vi "Read Admin Enable.vi"(4 "Close 2":bool, 8 "error in (no error)":errorcluster, 11 "Masterv2 in":refnum<class "Masterv2.lvclass">) -> (0 "error out":errorcluster, 1 "Boolean":bool, 3 "Masterv2 out":refnum<class "Masterv2.lvclass">, 5 "Admin Enable":bool, 6 "User Enable":bool, 7 "Programmer Enable":bool)   [LabVIEW 2014, in "Main Libraryv2.lvlib" / "Masterv2.lvclass"]
uses:
  Master/Masterv2.lvclass
panel:
  in  "DEL 2":bool
  in  "1 2":bool
  in  "2 2":bool
  in  "3 2":bool
  in  "4 2":bool
  in  "5 2":bool
  in  "6 2":bool
  in  "7 2":bool
  in  "8 2":bool
  in  "9 2":bool
  in  "0 2":bool
  in  "Enter 2":bool
  out "Login PWD 2":string
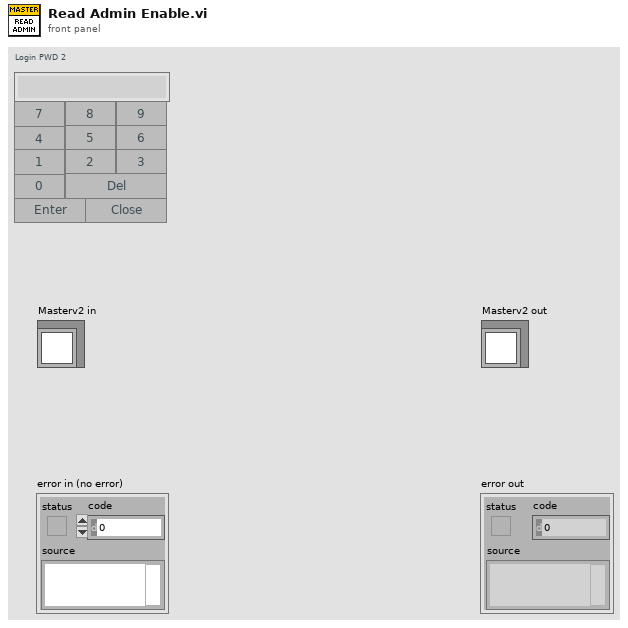
[diagram p1: front panel]
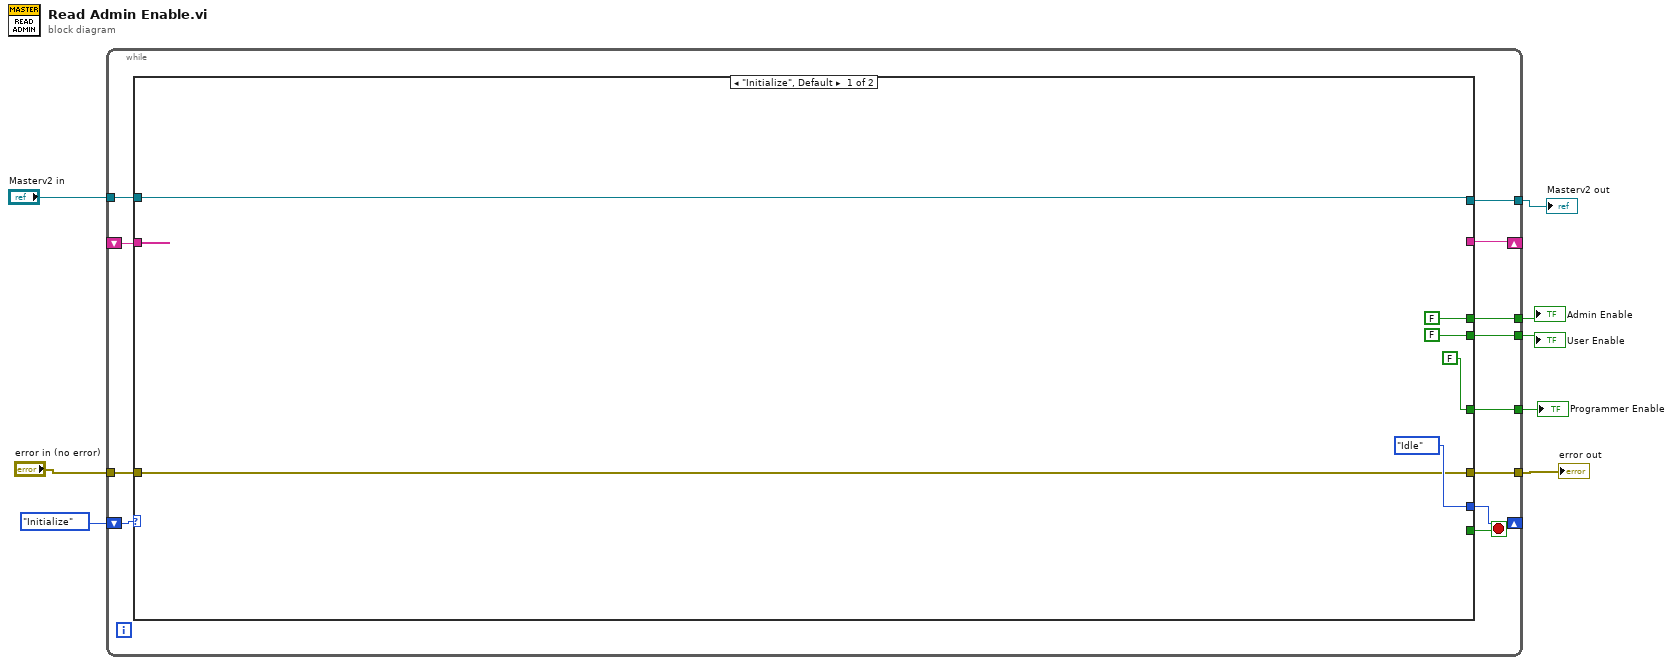
[diagram p0: block diagram]
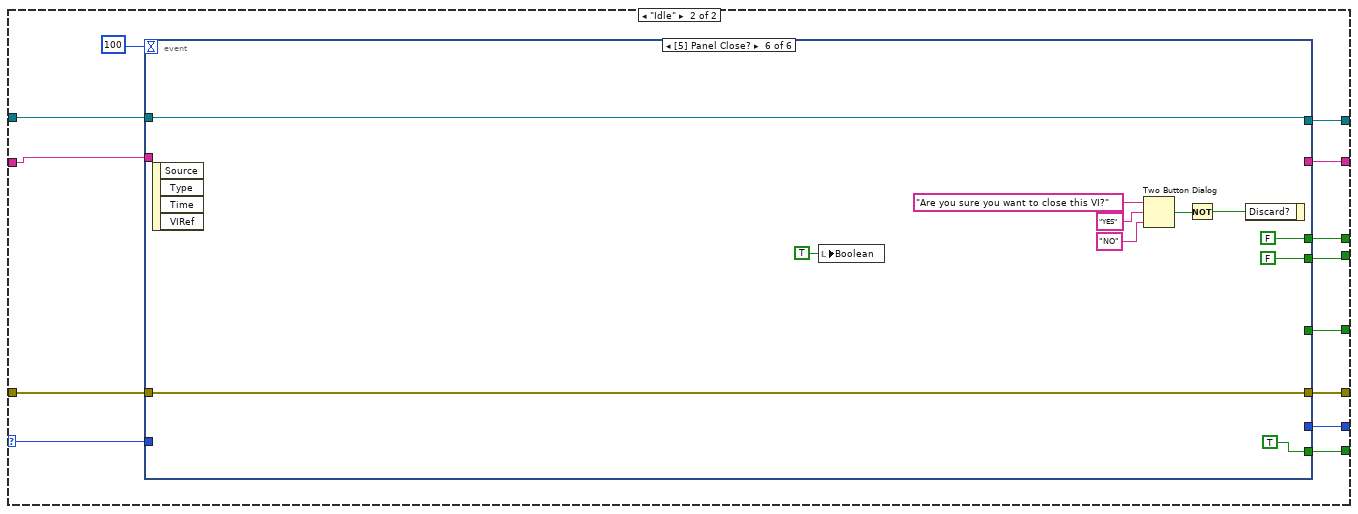
[diagram p2: hidden frame]
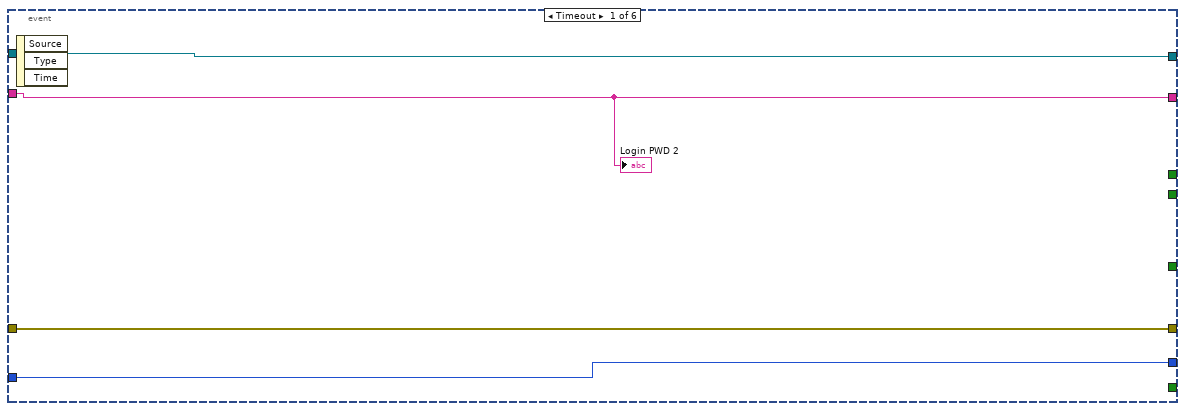
[diagram p3: hidden frame]
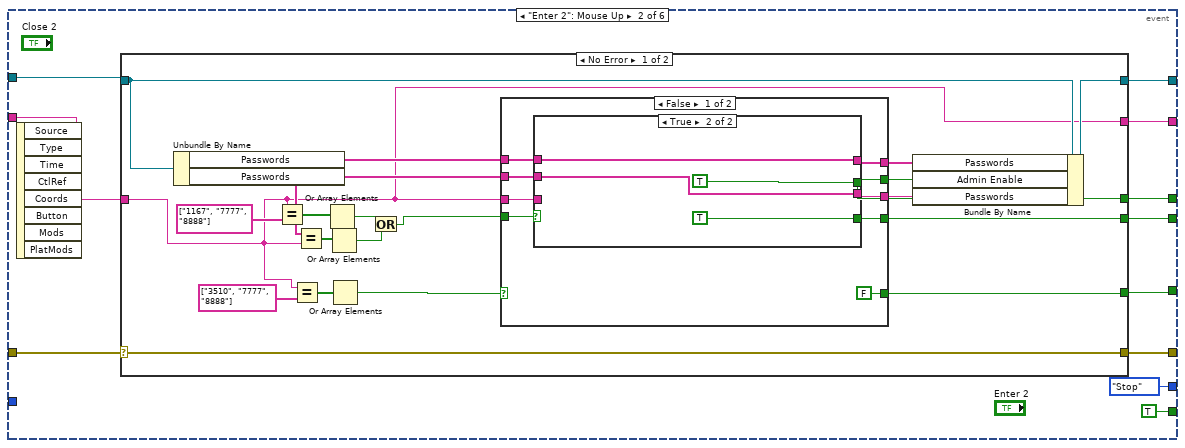
[diagram p4: hidden frame]
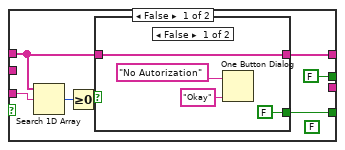
[diagram p5: hidden frame]
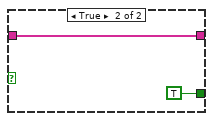
[diagram p6: hidden frame]
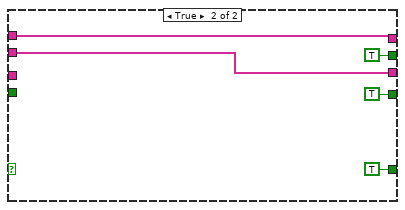
[diagram p7: hidden frame]
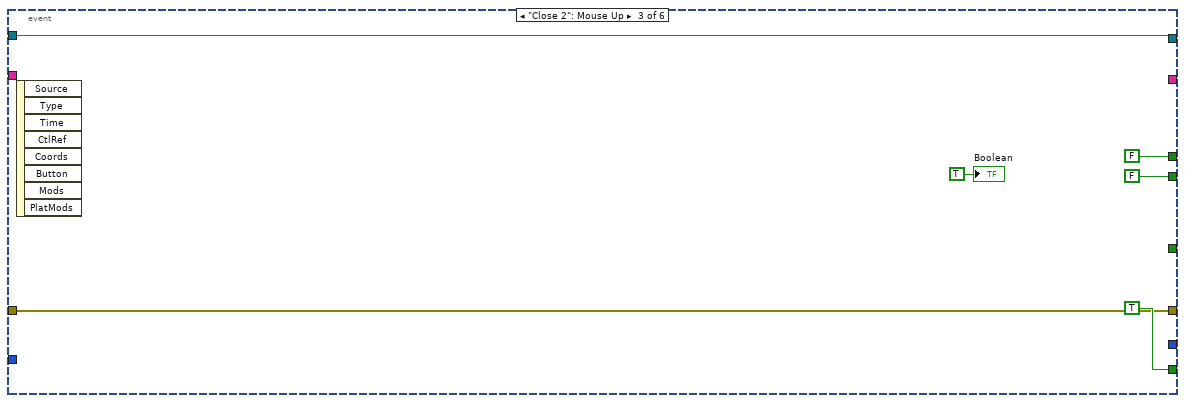
[diagram p9: hidden frame]
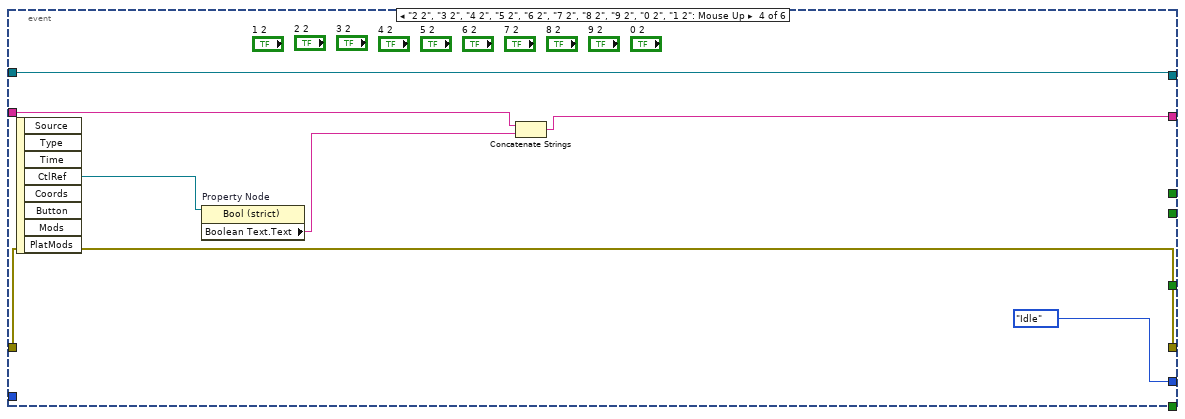
[diagram p10: hidden frame]
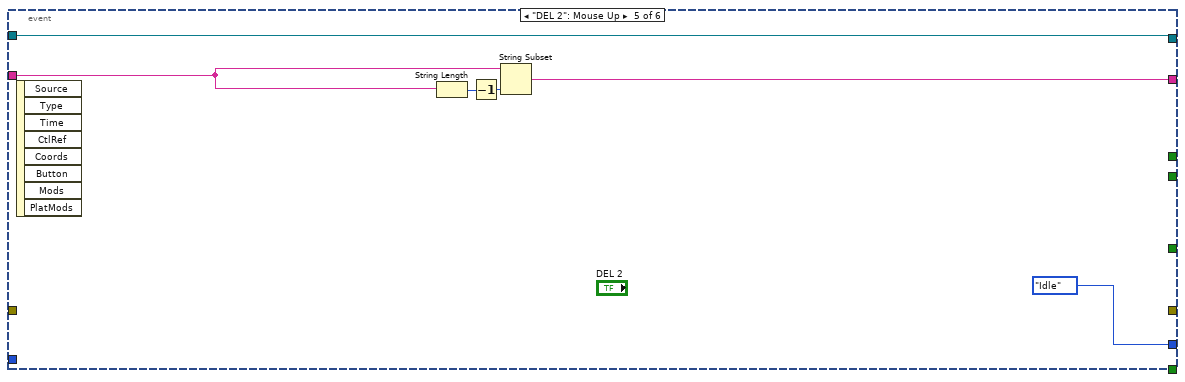
[diagram p11: hidden frame]
diagram:
  n1 = while {
    tunnel: "Masterv2 in" -> [w20]
    tunnel: "error in (no error)" -> [w19]
    tunnel: [w18] -> w2
    tunnel: [w17] -> w8
    tunnel: [w16] -> w7
    tunnel: [w15] -> w1
    shift-right: [w13] -> _
    shift-left: enum16{"Initialize", "Idle", "Stop"}."Initialize" -> [w14]
    shift-right: [w10] -> _
    shift-left: _ -> [w11]
    tunnel: [w9] -> w5
    stop <- w12 stop-if-true
    n2 = case shown="\"Initialize\", Default" w14 {
      selector: w14 -> [_ w32]
      tunnel: w20 -> [w24 w39]
      tunnel: w19 -> [w25 w38]
      tunnel: [w24 w37] -> w18
      tunnel: [FALSE ("Admin Enable") w36] -> w17
      tunnel: [FALSE ("User Enable") w35] -> w16
      tunnel: [w25 w34] -> w15
      tunnel: [enum16{"Initialize", "Idle", "Stop"}."Idle" w33] -> w13
      tunnel: [_ w31] -> w12
      tunnel: w11 -> [_ w28]
      tunnel: [_ w29] -> w10
      tunnel: [FALSE w27] -> w9
      frame "Initialize", Default {
      }
      frame "Idle" {
        n3 = event shown="[5] Panel Close?" {
          selector: _ -> [_ _ _ _ _ _]
          dyn-events: _ -> [_ _ _ _ _ _]
          timeout: 100 -> [_ _ _ _ _ _]
          tunnel: w39 -> [w42 w51 w110 w117 w123 w138]
          tunnel: w38 -> [w41 w50 w111 w116 _ w137]
          tunnel: [w42 w53 w110 w117 w123 w138] -> w37
          tunnel: [_ w49 FALSE ("Admin Enable") _ _ FALSE ("Admin Enable")] -> w36
          tunnel: [_ w48 FALSE ("User Enable") _ _ FALSE ("User Enable")] -> w35
          tunnel: [w41 w52 w111 w116 _ w137] -> w34
          tunnel: [w43 enum16{"Initialize", "Idle", "Stop"}."Stop" _ enum16{"Initialize", "Idle", "Stop"}."Idle" enum16{"Initialize", "Idle", "Stop"}."Idle" _] -> w33
          tunnel: w32 -> [w43 _ _ _ _ _]
          tunnel: [_ TRUE TRUE _ _ TRUE] -> w31
          tunnel: w28 -> [w40 w45 _ w119 w125 _]
          tunnel: [w40 w46 _ w118 w124 _] -> w29
          tunnel: [_ w44 _ _ _ _] -> w27
          event Timeout {
            n4 = event-data() -> ()  [unwired: 1 in, 3 out]
            "Login PWD 2" <- w40
          }
          event "Enter 2": Mouse Up {
            n5 = event-data() -> ()  [unwired: 1 in, 8 out]
            n6 = case shown="No Error" w50 {
              selector: w50 -> [w74 w108]
              tunnel: [w74 w108] -> w52
              tunnel: [w72 w107] -> w53
              tunnel: w51 -> [w73 w107]
              tunnel: [w71 _] -> w49
              tunnel: [w70 _] -> w48
              tunnel: w45 -> [w58 w106]
              tunnel: [w58 w106] -> w46
              tunnel: [w55 _] -> w44
              frame No Error {
                n7 = Unbundle By Name(w73) -> ("Passwords"=w69:string[], "Passwords"=w66:string[])
                n8 = Equal?(x=w58, y=string[] ["1167", "7777", "8888"] ("Setting Password.Passwords")) -> (x = y?=w62:bool[])
                n9 = Equal?(x=w58, y=string[] ["3510", "7777", "8888"] ("Setting Password.Passwords")) -> (x = y?=w57:bool[])
                n10 = Equal?(x=w66, y=w58) -> (x = y?=w61:bool[])
                n11 = Or Array Elements(Boolean array=w62) -> (logical OR=w60:bool)
                n12 = Or Array Elements(Boolean array=w61) -> (logical OR=w63:bool)
                n13 = Or Array Elements(Boolean array=w57) -> (logical OR=w56:bool)
                n14 = Or(x=w60, y=w63) -> (x .or. y?=w64:bool)
                n15 = case shown="False" w56 {
                  tunnel: [w83 TRUE ("Admin Enable")] -> w71
                  tunnel: [w82 TRUE ("User Enable")] -> w70
                  tunnel: w69 -> [w81 w105]
                  tunnel: [w80 w105] -> w68
                  tunnel: w66 -> [w79 w104]
                  tunnel: [w78 w104] -> w65
                  tunnel: w64 -> [w77 _]
                  tunnel: w58 -> [w76 _]
                  tunnel: [FALSE TRUE] -> w55
                  frame False {
                    n16 = case shown="True" w77 {
                      tunnel: [w90 w100] -> w80
                      tunnel: w81 -> [w89 w100]
                      tunnel: [FALSE ("Admin Enable") TRUE ("Admin Enable")] -> w83
                      tunnel: [w85 TRUE ("User Enable")] -> w82
                      tunnel: w76 -> [w84 _]
                      tunnel: w79 -> [_ w97]
                      tunnel: [_ w97] -> w78
                      frame False {
                        (unwired) FALSE
                        n17 = Search 1D Array(1D array=w89, element=w84) -> (index of element=w88:i32)  [unwired: 1 in]
                        n18 = Greater Or Equal To 0?(x=w88) -> (x >= 0?=w87:bool)
                        n19 = case shown="False" w87 {
                          tunnel: [w94 w96] -> w90
                          tunnel: w89 -> [w94 w96]
                          tunnel: [FALSE ("User Enable") TRUE ("User Enable")] -> w85
                          frame False {
                            n20 = One Button Dialog(message="No Autorization", button name ("OK")="Okay") -> ()  [unwired: 1 out]
                          }
                          frame True {
                          }
                        }
                      }
                      frame True {
                      }
                    }
                  }
                  frame True {
                  }
                }
                n21 = Bundle By Name(cluster=w73, "Passwords"=w68, "Admin Enable"=w71, "Passwords"=w65) -> (w72:refnum<class "Masterv2.lvclass">)
              }
              frame Error {
              }
            }
          }
          event "Close 2": Mouse Up {
            n22 = event-data() -> ()  [unwired: 1 in, 8 out]
            "Boolean" <- TRUE ("Boolean")
          }
          event "2 2", "3 2", "4 2", "5 2", "6 2", "7 2", "8 2", "9 2", "0 2", "1 2": Mouse Up {
            n23 = event-data() -> ("CtlRef"=w120:refnum<vi>)  [unwired: 1 in, 7 out]
            n24 = property on="Property Node" class="Bool (strict)"(reference=w120) -> ("Boolean Text.Text"=w121:string)  [unwired: 1 in, 2 out]
            n25 = Concatenate Strings(w119, w121) -> (w118:string)
          }
          event "DEL 2": Mouse Up {
            n26 = event-data() -> ()  [unwired: 1 in, 8 out]
            n27 = String Length(string=w125) -> (length=w127:i32)
            n28 = Decrement(x=w127) -> (x-1=w126:i32)
            n29 = String Subset(string=w125, length (rest)=w126) -> (substring=w124:string)  [unwired: 1 in]
          }
          event Panel Close? {
            n30 = event-data() -> ()  [unwired: 1 in, 4 out]
            n31 = local write "Boolean"(TRUE ("Boolean")) -> ()
            n32 = Two Button Dialog(message="Are you sure you want to close this VI?", 1:"NO" ("F button name (\"Cancel\")"), 2:"YES" ("T button name (\"OK\")")) -> (T button?=w134:bool)
            n33 = Not(x=w134) -> (.not. x?=w133:bool)
            n34 = event-data("Discard?"=w133) -> ()  [unwired: 1 in, 1 out]
          }
        }
      }
    }
  }
  "error out" <- w1
  "Masterv2 out" <- w2
  "Admin Enable" <- w8
  "User Enable" <- w7
  "Programmer Enable" <- w5
